vi "enmu_sub.vi"(10 "Enum":enum16{"Team A", "Team B", "Team C"}(ring)) -> ()   [LabVIEW 2021]
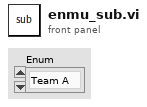
[diagram p1: front panel]
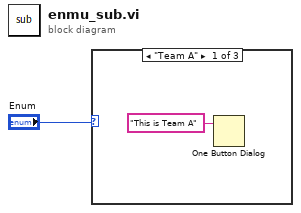
[diagram p0: block diagram]
diagram:
  n1 = case shown="\"Team A\"" "Enum" {
    frame "Team A" {
      n2 = One Button Dialog(message="This is Team A") -> ()  [unwired: 1 in, 1 out]
    }
    frame "Team B" {
    }
    frame "Team C" {
    }
  }
